vi "INIT.vi"(8 "error in (no error)":errorcluster, 11 "OWIS_TANGO in":refnum<class "OWIS_TANGO.lvclass">) -> (0 "error out":errorcluster, 3 "OWIS_TANGO out":refnum<class "OWIS_TANGO.lvclass">)   [LabVIEW 2020, in "OWIS_TANGO.lvclass"]
uses:
  OWIS_TANGO.lvclass
  C:/dev/TRANCON/Classes/GeneralFunctionality/GeneralFunctionality.lvclass
  GeneralFunctionality/GeneralFunctionality.lvclass/GeneralFunctionality.ctl
  GeneralFunctionality/GeneralFunctionality.lvclass
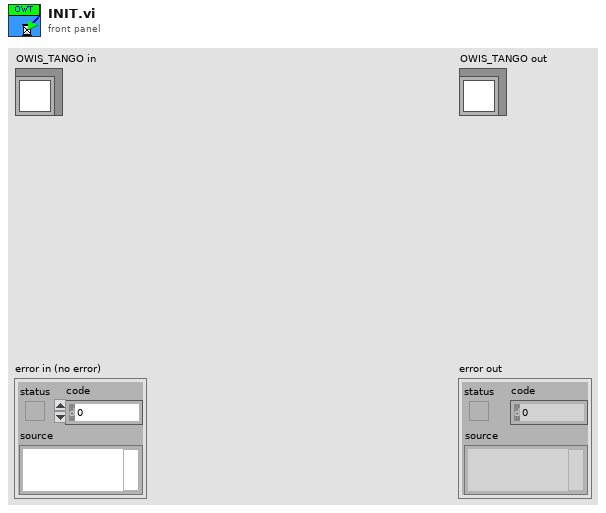
[diagram p1: front panel]
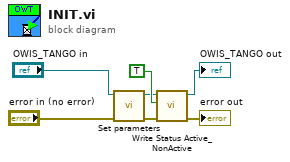
[diagram p0: block diagram]
diagram:
  n1 = call-dynamic "Set parameters.vi"("error in (no error)"="error in (no error)", "OWIS_TANGO en entrée"="OWIS_TANGO in") -> ("error out"=w4:errorcluster, "OWIS_TANGO en sortie"=w3:refnum<class "OWIS_TANGO.lvclass">)  [unwired: 8 in]
  n2 = call "Write Status Active_NonActive.vi"("error in (no error)"=w4, "Status Active/NonActive"=TRUE, "GeneralFunctionality in"=w3) -> ("error out"=→"error out":errorcluster, "GeneralFunctionality out"=→"OWIS_TANGO out":refnum<class "OWIS_TANGO.lvclass">)  [unwired: 7 in]
